vi "Get Alias.vi"(8 "error in (no error)":errorcluster, 11 "Data in":refnum<class "Data.lvclass">) -> (0 "error out":errorcluster, 2 "Alias":string, 3 "Data out":refnum<class "Data.lvclass">)   [LabVIEW 2020, in "Data.lvlib" / "Data.lvclass"]
doc: "Return the Alias of the Data class.\nThe default implmentation returns the base class name."
uses:
  Data.lvclass
  <vilib>/Utility/LVClass/Get LV Class Name.vi
  Data.lvlib
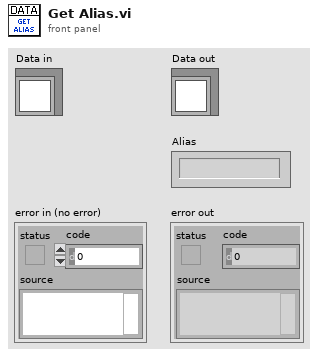
[diagram p1: front panel]
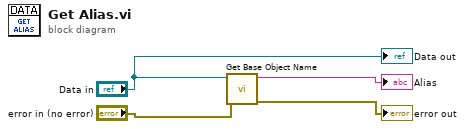
[diagram p0: block diagram]
diagram:
  n1 = call "Get Base Object Name.vi"("error in (no error)"="error in (no error)", "Object in"="Data in") -> ("error out"=→"error out":errorcluster, "Base class name"=→"Alias":string)  [unwired: 8 in]
  "Data out" <- "Data in"
